vi "lookupElement.vi"(8 "error in (no error)":errorcluster, 9 "lookupIn":string, 10 "lookupElement":string, 11 "ICSettingsViewer in":refnum<class "ICSettingsViewer.lvclass">) -> (0 "error out":errorcluster, 2 "element":string, 3 "ICSettingsViewer out":refnum<class "ICSettingsViewer.lvclass">)   [LabVIEW 2011, in "Views.lvlib" / "Camera.lvlib" / "ICSettingsViewer.lvclass"]
uses:
  ICSettingsViewer.lvclass
  Tools/SettingsEventManager/SettingsEventsManager.lvclass
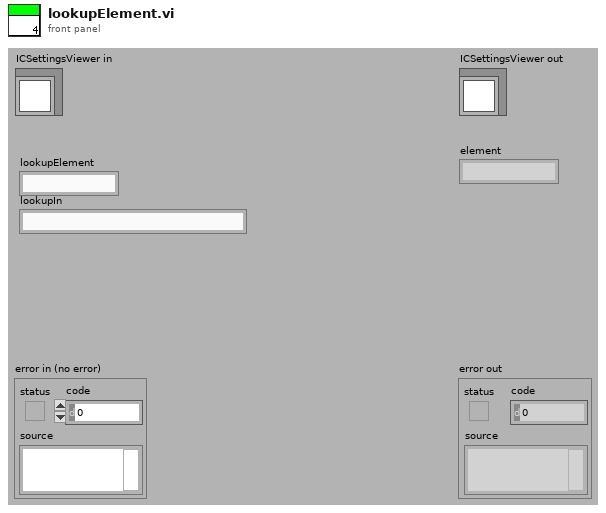
[diagram p1: front panel]
types:
  T1 = enum16{"Number", "String", "NumberArray", "StringArray", "xmlNode"}
  T2 = cluster{"settingsFrontEndEvents":cluster{"loadSettingsFromPath":refnum<user-event>, "lookUpElementEvent":refnum<user-event>, "saveSettings":refnum<user-event>, "loadSettings":refnum<user-event>, "close":refnum<user-event>, "replaceElement":refnum<user-event>, "findParentNodes":refnum<user-event>, "createNode":refnum<user-event>}, "settingBackEndEvents":cluster{"defaultSettingsPathRequest":refnum<user-event>, "searchResultEvent":refnum<user-event>, "settingsSaved":refnum<user-event>, "settingsLoaded":refnum<user-event>, "foundParentNode":refnum<user-event>}}
  T3 = cluster{"lookupElement":string, "lookupIn":string, "typeEnum":enum16{"Number", "String", "NumberArray", "StringArray", "xmlNode"}}
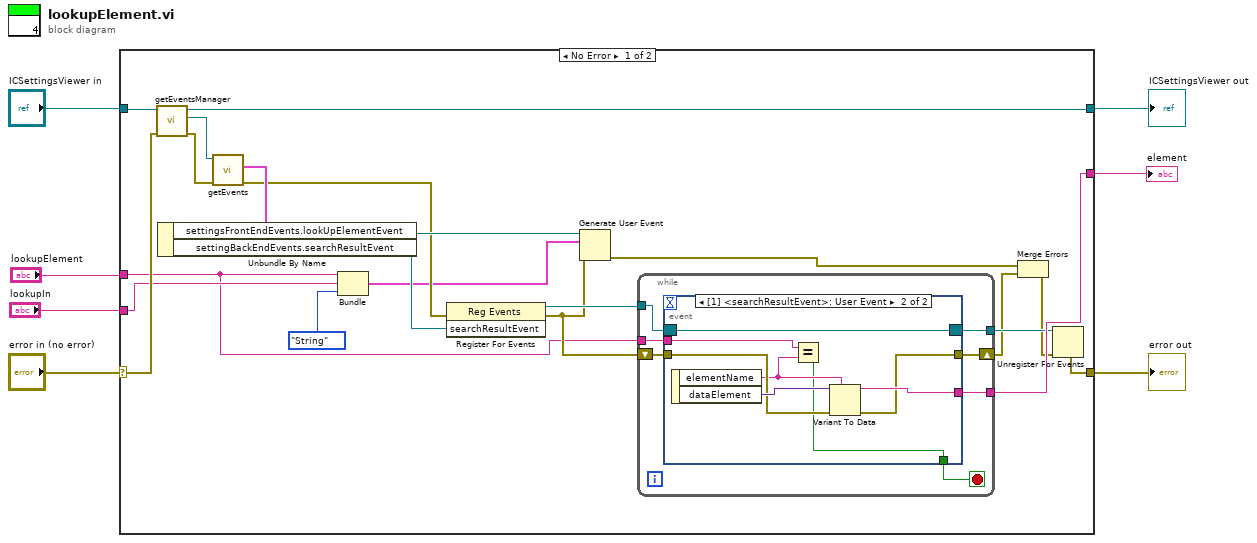
[diagram p0: block diagram]
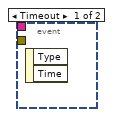
[diagram p2: hidden frame]
diagram:
  n1 = case shown="No Error" "error in (no error)" {
    selector: "error in (no error)" -> [w24 w45]
    tunnel: [w12 w45] -> w6
    tunnel: [w25 w44] -> w4
    tunnel: "ICSettingsViewer in" -> [w26 w44]
    tunnel: "lookupElement" -> [w8 _]
    tunnel: "lookupIn" -> [w17 _]
    tunnel: [w14 _] -> w1
    frame No Error {
      n2 = call-dynamic "getEventsManager.vi"("error in (no error)"=w24, "SettingsViewer.lvclass in"=w26) -> ("error out"=w27:errorcluster, "Tools.lvlib:Settings.lvlib:SettingsEventsManager.lvclass"=w28:refnum<class "SettingsEventsManager.lvclass">, "SettingsViewer.lvclass out"=w25:refnum<class "ICSettingsViewer.lvclass">)  [unwired: 7 in]
      n3 = call-dynamic "getEvents.vi"("error in (no error)"=w27, "SettingsEventsManager in"=w28) -> ("error out"=w20:errorcluster, "settingsEvents"=w23:T2)  [unwired: 7 in, 1 out]
      n4 = Unbundle By Name(w23) -> ("settingsFrontEndEvents.lookUpElementEvent"=w22:refnum<user-event>, "settingBackEndEvents.searchResultEvent"=w21:refnum<user-event>)
      n5 = Bundle("lookupElement"=w8, "lookupIn"=w17, "typeEnum"=T1."String") -> (w15:T3)  [unwired: 1 in]
      n6 = register-events(error in=w20, w21) -> (reference out=w19:refnum<event-registration>, error out=w18:errorcluster)  [unwired: 1 in]
      n7 = Generate User Event(user event=w22, event data cluster=w15, error in=w18) -> (error out=w11:errorcluster)  [unwired: 1 out]
      n8 = while {
        tunnel: w19 -> [w35]
        shift-right: [w32] -> w10
        shift-left: w18 -> [w34]
        tunnel: [w33] -> w14
        tunnel: [w31] -> w13
        tunnel: w8 -> [w29]
        stop <- w30 stop-if-true
        n9 = event shown="[1] <searchResultEvent>: User Event" {
          selector: w35 -> [_ w39]
          dyn-events: [_ w39] -> w31
          timeout: _ -> [_ _]
          tunnel: w34 -> [_ w42]
          tunnel: [_ w41] -> w33
          tunnel: [_ w40] -> w32
          tunnel: [_ w36] -> w30
          tunnel: w29 -> [_ w38]
          event Timeout {
            n10 = event-data() -> ()  [unwired: 1 in, 2 out]
          }
          event User Event {
            n11 = event-data() -> ("elementName"=w37:string, "dataElement"=w43:variant)  [unwired: 1 in]
            n12 = Equal?(x=w38, y=w37) -> (x = y?=w36:bool)
            n13 = Variant To Data(error in=w42, type=w37, Variant=w43) -> (data=w41:string, error out=w40:errorcluster)
          }
        }
      }
      n14 = Merge Errors(w11, w10) -> (w9:errorcluster)
      n15 = Unregister For Events(event registration refnum=w13, error in=w9) -> (error out=w12:errorcluster)
    }
    frame Error {
    }
  }
  "error out" <- w6
  "ICSettingsViewer out" <- w4
  "element" <- w1
